vi "TwTof2Mass.vi"(1 "p":dbl[](array[numeric]), 2 "MassCalibMode":i32, 3 "TofSample":dbl) -> (0 "mass":dbl)   [LabVIEW 2009]
uses:
  TwToolDll.dll
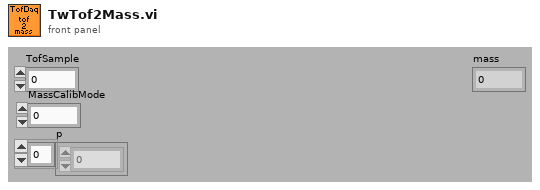
[diagram p1: front panel]
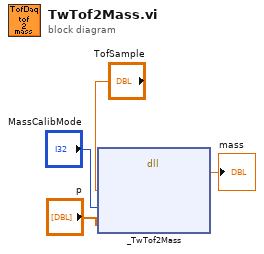
[diagram p0: block diagram]
diagram:
  n1 = dll-call lib="C:/src/TofDaq/APIandWrappers/LabView/TwToolDll/TwToolDll.dll" fn="_TwTof2Mass"("TofSample"="TofSample", "MassCalibMode"="MassCalibMode", "p"="p") -> ("mass"=→"mass":dbl)  [unwired: 6 in, 2 out]
